vi "zs_parser.vi"() -> ()   [LabVIEW 2014, in "Dialogue.lvlib" / "Dialogue.lvclass"]
uses:
  Dialogue_lib/DialogueActor/Dialogue.lvclass
  ctl/Point.ctl
panel:
  out "goal_with_force_array":T1(array[cluster])
  out "数值":dbl
  out "机器人语音指令数据簇数组(Voice)":T2(array[cluster])
  out "连接的字符串":string
  out "连接的字符串 2":string
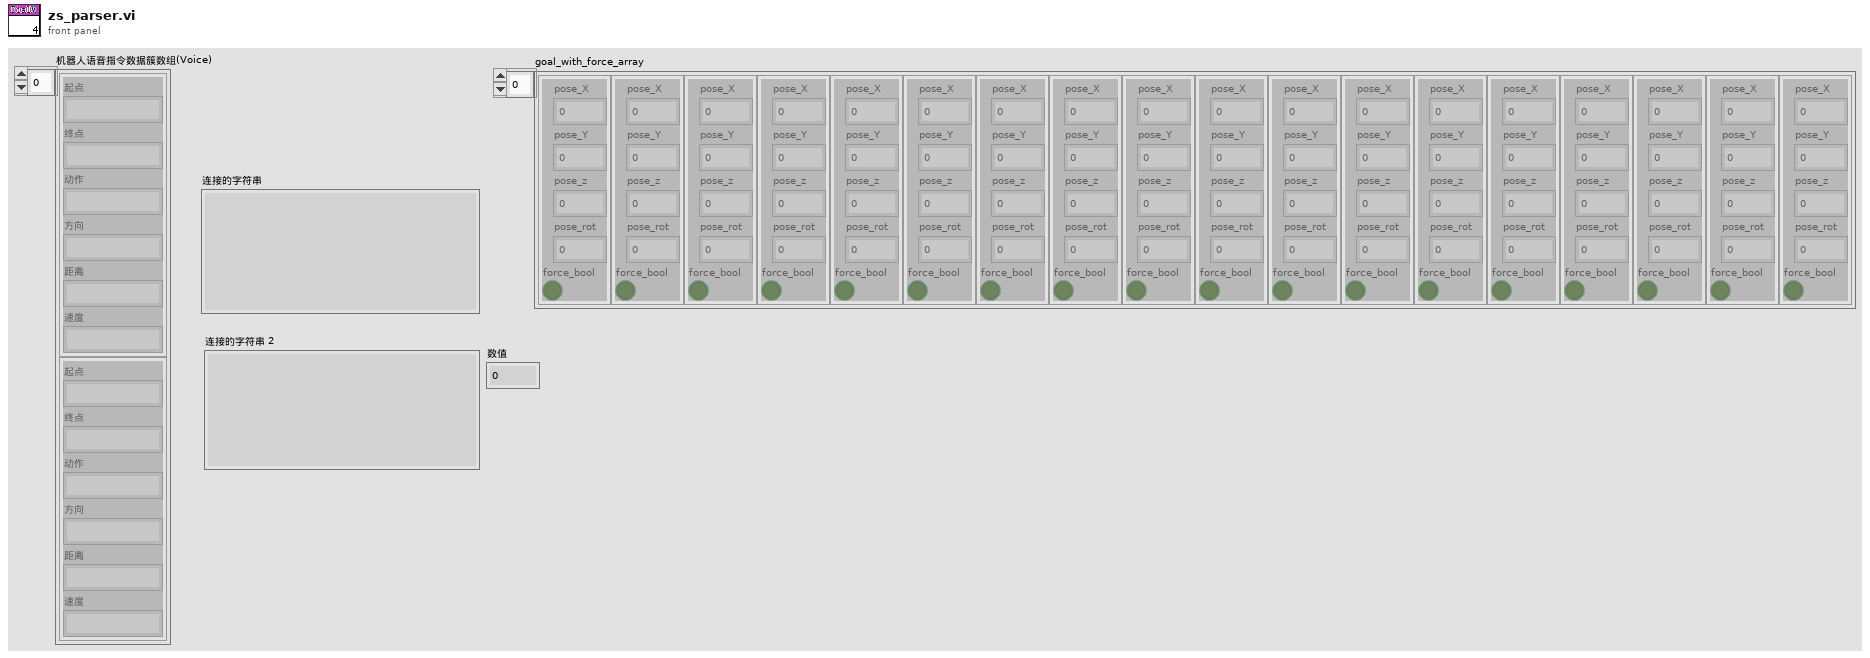
[diagram p1: front panel]
types:
  T1 = cluster{"pose_X":dbl, "pose_Y":dbl, "pose_z":dbl, "pose_rot":dbl, "force_bool":bool}[]
  T2 = cluster{"起点":string, "终点":string, "动作":string, "方向":string, "距离":string, "速度":string}[]
  T3 = typedef "Point.ctl" = cluster{"x":dbl, "y":dbl, "z":dbl}
  T4 = cluster{"pose_X":dbl, "pose_Y":dbl, "pose_z":dbl, "pose_rot":dbl, "force_bool":bool}
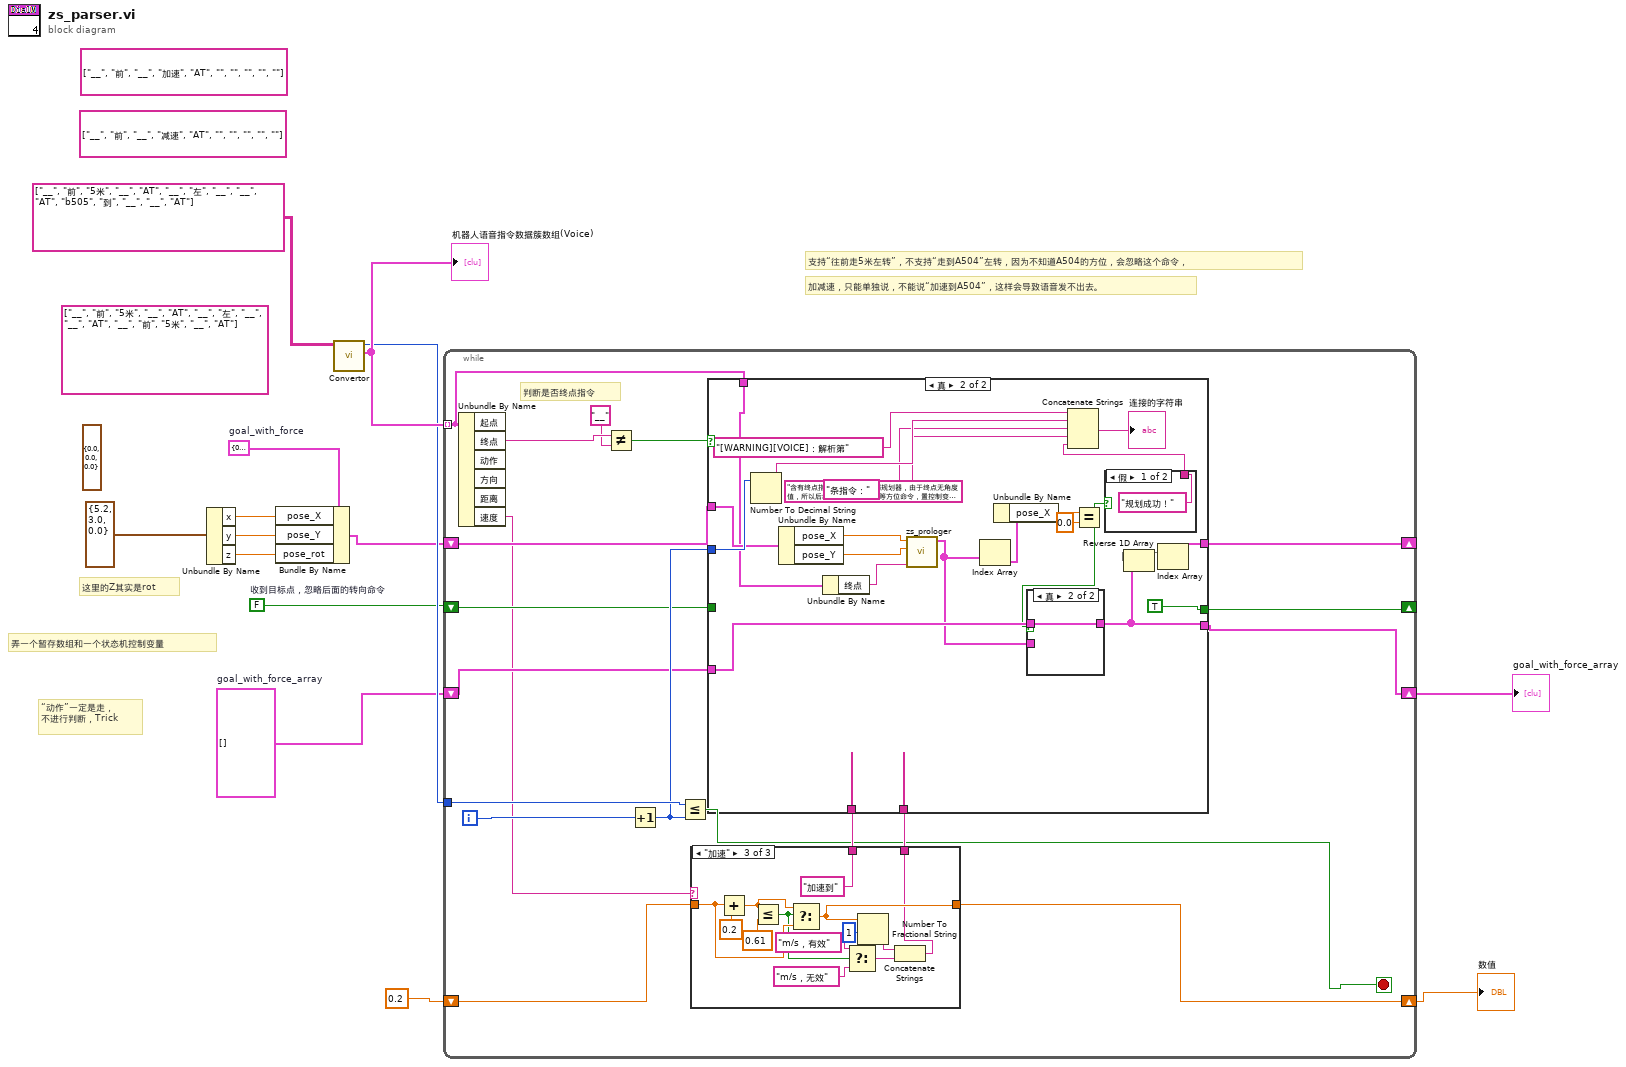
[diagram p0: block diagram]
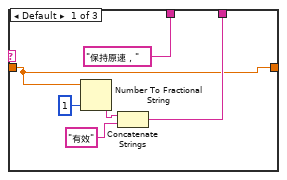
[diagram p2: hidden frame]
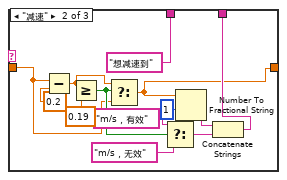
[diagram p3: hidden frame]
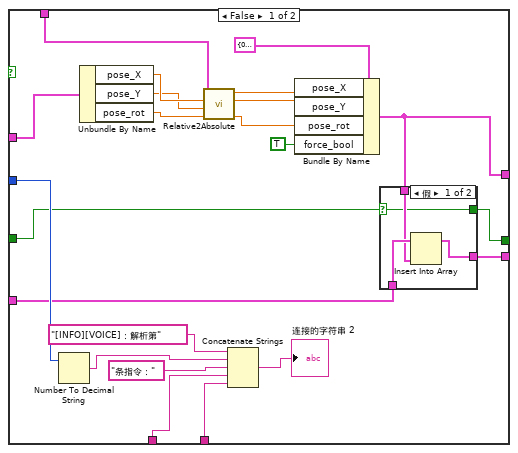
[diagram p4: hidden frame]
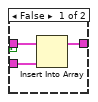
[diagram p6: hidden frame]
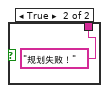
[diagram p7: hidden frame]
diagram:
  (unwired) string[][] [["__", "前", "5米", "__", "AT"], ["__", "左", "__", "__", "AT"], ["__", "前", "5米", "__", "AT"]] ("格式化机器人指令 2")
  w4 = T4 {"pose_X"=0.0, "pose_Y"=0.0, "pose_z"=0.0, "pose_rot"=0.0, "force_bool"=FALSE}  # goal_with_force
  w5 = T1 []  # goal_with_force_array
  w6 = FALSE  # 收到目标点，忽略后面的转向命令
  (unwired) string[][] [["__", "前", "__", "加速", "AT"], ["", "", "", "", ""]] ("格式化机器人指令 2")
  (unwired) string[][] [["__", "前", "__", "减速", "AT"], ["", "", "", "", ""]] ("格式化机器人指令 2")
  (unwired) T3 {"x"=0.0, "y"=0.0, "z"=0.0} ("值(信号)")
  # "加减速，只能单独说，不能说“加速到A504”，这样会导致语音发不出去。"
  # "这里的Z其实是rot"
  # "支持“往前走5米左转”，不支持“走到A504”左转，因为不知道A504的方位，会忽略这个命令，"
  # "弄一个暂存数组和一个状态机控制变量"
  # "“动作”一定是走，\n不进行判断，Trick"
  n1 = Unbundle By Name(T3 {"x"=5.2, "y"=3.0, "z"=0.0} ("值(信号)")) -> ("x"=w10:dbl, "y"=w9:dbl, "z"=w8:dbl)
  n2 = Bundle By Name(cluster=w4, "pose_X"=w10, "pose_Y"=w9, "pose_rot"=w8) -> (w7:T4)
  n3 = call "Convertor.vi"("格式化机器人指令"=string[][] [["__", "前", "5米", "__", "AT"], ["__", "左", "__", "__", "AT"], ["b505", "到", "__", "__", "AT"]] ("格式化机器人指令 2")) -> ("机器人语音指令数据簇数组(Voice)"=w14:T2, "命令个数"=w13:i32)  [unwired: 8 in, 1 out]
  "机器人语音指令数据簇数组(Voice)" <- w14
  n4 = while {
    tunnel: w14 -> [w32] mode=indexing
    shift-right: [w21] -> _
    shift-left: w7 -> [w23]
    tunnel: w13 -> [w30]
    shift-right: [w26] -> w11
    shift-left: 0.2 -> [w28]
    shift-right: [w18] -> w3
    shift-left: w5 -> [w22]
    shift-right: [w19] -> _
    shift-left: w6 -> [w20]
    i -> [w31]
    stop <- w24 stop-if-true
    # "判断是否终点指令"
    n5 = Unbundle By Name(w32) -> ("终点"=w33:string, "速度"=w17:string)  [unwired: 4 out]
    n6 = Not Equal?(x=w33, y="__") -> (x != y?=w15:bool)
    n7 = Increment(x=w31) -> (x+1=w29:i32)
    n8 = Less Or Equal?(x=w30, y=w29) -> (x <= y?=w24:bool)
    n9 = case shown="\"加速\"" w17 {
      tunnel: w28 -> [w35 w41 w61]
      tunnel: ["保持原速，" ("Event Text") "想减速到" ("Event Text") "加速到" ("Event Text")] -> w27
      tunnel: [w35 w42 w56] -> w26
      tunnel: [w36 w43 w55] -> w25
      frame Default {
        n10 = Number To Fractional String(number=w35, precision (6)=i16 1 ("精度(6)")) -> (F-format string=w38:string)  [unwired: 2 in]
        n11 = Concatenate Strings(w38, "有效" ("Event Text")) -> (w36:string)
      }
      frame "减速" {
        n12 = Subtract(x=w41, y=0.2) -> (x-y=w50:dbl)
        n13 = Greater Or Equal?(x=w50, y=0.19) -> (x >= y?=w49:bool)
        n14 = Select(t=w50, s=w49, f=w41) -> (s? t:f=w42:dbl)
        n15 = Select(t="m/s，有效" ("Event Text"), s=w49, f="m/s，无效" ("Event Text")) -> (s? t:f=w46:string)
        n16 = Number To Fractional String(number=w42, precision (6)=i16 1 ("精度(6)")) -> (F-format string=w45:string)  [unwired: 2 in]
        n17 = Concatenate Strings(w45, w46) -> (w43:string)
      }
      frame "加速" {
        n18 = Add(x=w61, y=0.2) -> (x+y=w62:dbl)
        n19 = Less Or Equal?(x=w62, y=0.61) -> (x <= y?=w54:bool)
        n20 = Select(t=w62, s=w54, f=w61) -> (s? t:f=w56:dbl)
        n21 = Select(t="m/s，有效" ("Event Text"), s=w54, f="m/s，无效" ("Event Text")) -> (s? t:f=w58:string)
        n22 = Number To Fractional String(number=w56, precision (6)=i16 1 ("精度(6)")) -> (F-format string=w57:string)  [unwired: 2 in]
        n23 = Concatenate Strings(w57, w58) -> (w55:string)
      }
    }
    n24 = case shown="真" w15 {
      tunnel: w32 -> [w87 w106]
      tunnel: [w71 w100] -> w21
      tunnel: w23 -> [w79 w109]
      tunnel: w29 -> [w83 w115]
      tunnel: w27 -> [w81 _]
      tunnel: w25 -> [w80 _]
      tunnel: w22 -> [w72 w104]
      tunnel: [w67 w102] -> w18
      tunnel: w20 -> [w69 _]
      tunnel: [w68 TRUE] -> w19
      frame False {
        n25 = Number To Decimal String(number=w83) -> (decimal integer string=w85:string)  [unwired: 1 in]
        n26 = Unbundle By Name(w79) -> ("pose_X"=w78:dbl, "pose_Y"=w77:dbl, "pose_rot"=w76:dbl)
        n27 = call "Relative2Absolute.vi"("机器人语音指令数据簇"=w87, "now_pose_X"=w78, "now_pose_Y"=w77, "now_pose_Rot_deg"=w76) -> ("x"=w75:dbl, "y"=w74:dbl, "Rot_deg"=w73:dbl)  [unwired: 4 in]
        n28 = Concatenate Strings("[INFO][VOICE]：解析第" ("Event Text"), w85, "条指令：" ("Event Text"), w81, w80) -> (→"连接的字符串 2":string)
        n29 = Bundle By Name(cluster=T4 {"pose_X"=0.0, "pose_Y"=0.0, "pose_z"=0.0, "pose_rot"=0.0, "force_bool"=FALSE} ("goal_with_force"), "pose_X"=w75, "pose_Y"=w74, "pose_rot"=w73, "force_bool"=TRUE) -> (w71:T4)
        n30 = case shown="假" w69 {
          selector: w69 -> [w89 w93]
          tunnel: w72 -> [w91 w92]
          tunnel: w71 -> [w90 _]
          tunnel: [w89 w93] -> w68
          tunnel: [w88 w92] -> w67
          frame False {
            n31 = Insert Into Array(array=w91, new element=w90) -> (w88:T1)  [unwired: 1 in]
          }
          frame True {
          }
        }
      }
      frame True {
        n32 = Number To Decimal String(number=w115) -> (decimal integer string=w113:string)  [unwired: 1 in]
        n33 = Unbundle By Name(w109) -> ("pose_X"=w108:dbl, "pose_Y"=w107:dbl)
        n34 = Unbundle By Name(w106) -> ("终点"=w105:string)
        n35 = call "zs_prologer.vi"("node_goal"=w105, "y"=w107, "x"=w108) -> ("goal_array"=w99:T1)  [unwired: 7 in]
        n36 = Index Array(array=w99) -> (element=w98:T4)  [unwired: 1 in]
        n37 = Unbundle By Name(w98) -> ("pose_X"=w97:dbl)
        n38 = Equal?(x=w97, y=0.0) -> (x = y?=w94:bool)
        n39 = case shown="真" w94 {
          tunnel: w104 -> [w118 w119]
          tunnel: [w117 w119] -> w102
          tunnel: w99 -> [w116 _]
          frame False {
            n40 = Insert Into Array(array=w118, new element=w116) -> (w117:T1)  [unwired: 1 in]
          }
          frame True {
          }
        }
        n41 = case shown="假" w94 {
          tunnel: ["规划成功！" "规划失败！"] -> w95
          frame False {
          }
          frame True {
          }
        }
        n42 = Concatenate Strings("[WARNING][VOICE]：解析第" ("Event Text"), w113, "条指令：" ("Event Text"), "含有终点指令元素，调用全局规划器，由于终点无角度值，所以后续无法执行“左转”等方位命令，置控制变量，忽略此“转向命令”\n" ("Event Text"), w95) -> (→"连接的字符串":string)
        n43 = Reverse 1D Array(array=w102) -> (reversed array=w101:T1)
        n44 = Index Array(array=w101) -> (element=w100:T4)  [unwired: 1 in]
      }
    }
  }
  "数值" <- w11
  "goal_with_force_array" <- w3
